vi "G#Object_RegisterExternalCreateProcessCallers.vi"(1 "Action":T1(ring), 5 "error in (no error)":errorcluster) -> (15 "StopExternalCreate?":bool, 19 "error out":errorcluster)   [LabVIEW 2020, in "G#Object.lvclass"]
doc: "Registers or deregister top-level callesrs."
uses:
  G#Object.lvclass
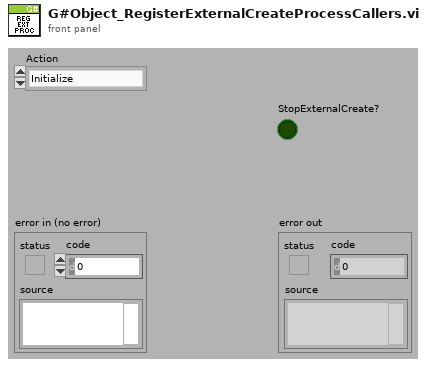
[diagram p1: front panel]
types:
  T1 = enum16{"Initialize", "Register", "Unregister", "Clear"}
  T2 = enum32{"Bad", "Idle", "Run top level", "Running"}
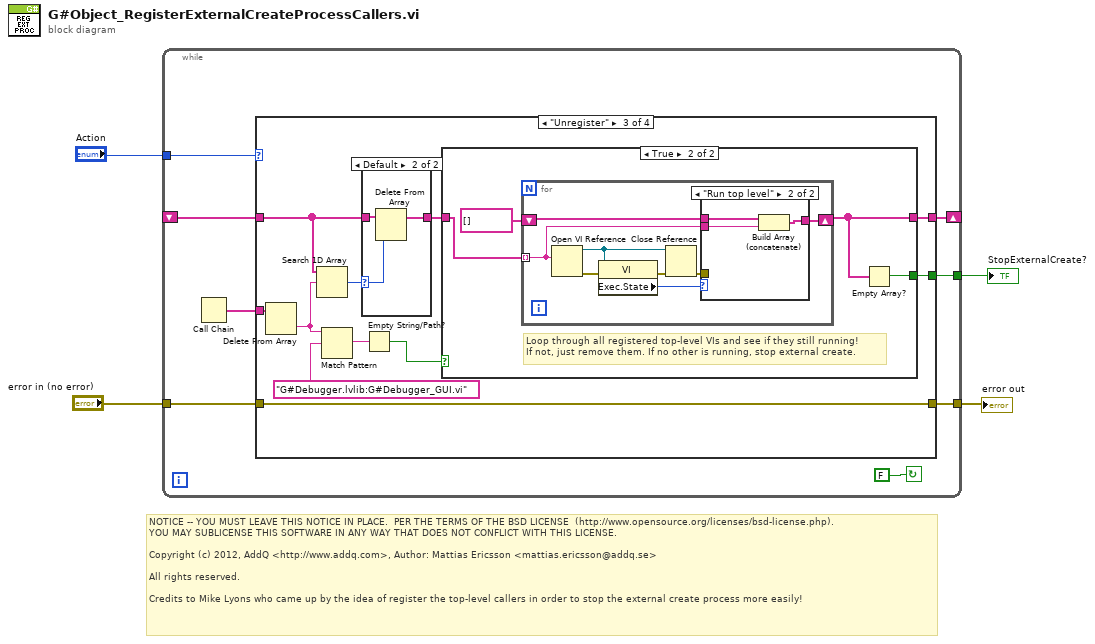
[diagram p0: block diagram]
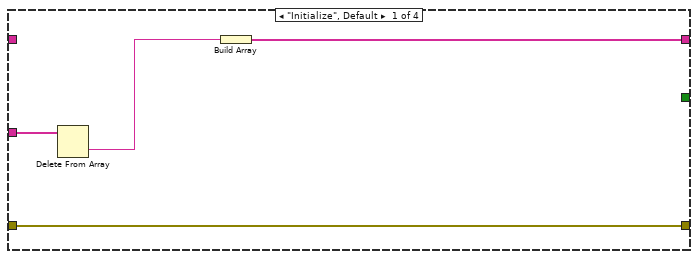
[diagram p2: hidden frame]
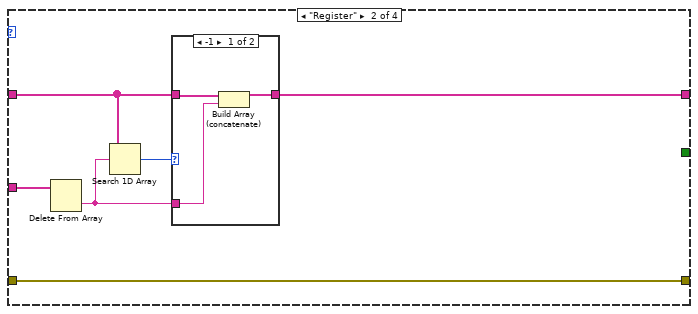
[diagram p3: hidden frame]
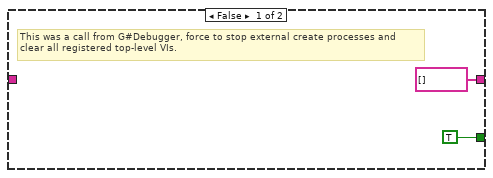
[diagram p5: hidden frame]
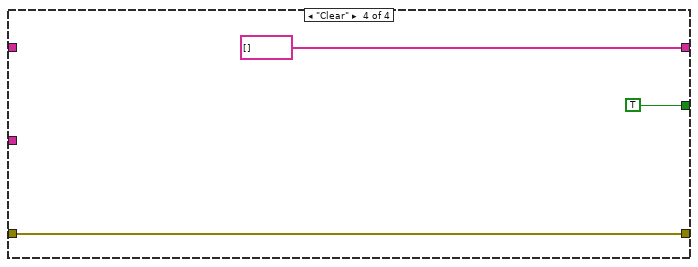
[diagram p8: hidden frame]
diagram:
  # "NOTICE -- YOU MUST LEAVE THIS NOTICE IN PLACE.  PER THE TERMS OF THE BSD LICENSE  (http://www.opensource.org/licenses/bsd-license.php).\nYOU MAY SUBLICENSE THIS SOFTWARE IN ANY WAY THAT DOES NOT CONFLICT WITH THIS LICENSE.\n\nCopyright (c) 2012, AddQ <http://www.addq.com>, Author: Mattias Ericsson <mattias.ericsson@addq.se>\n\nAll rights reserved.\n\nCredits to Mike Lyons who came up by the idea of register the top-level callers in order to stop the external create process more easily!"
  n1 = while {
    tunnel: "error in (no error)" -> [w11]
    tunnel: "Action" -> [w12]
    shift-right: [w8] -> _
    shift-left: _ -> [w6]
    tunnel: [w7] -> w2
    tunnel: [w5] -> w1
    stop <- FALSE continue-if-true
    n2 = Call Chain() -> (call chain=w9:string[])
    n3 = case shown="\"Unregister\"" w12 {
      tunnel: w11 -> [w13 w17 w33 w61]
      tunnel: w9 -> [w16 w22 w37 _]
      tunnel: [w15 w19 w31 string[] []] -> w8
      tunnel: [w13 w17 w33 w61] -> w7
      tunnel: w6 -> [_ w20 w35 _]
      tunnel: [_ _ w32 TRUE] -> w5
      frame "Initialize", Default {
        n4 = Delete From Array(array=w16) -> (deleted portion=w14:string)  [unwired: 2 in, 1 out]
        n5 = Build Array(w14) -> (w15:string[])
      }
      frame "Register" {
        n6 = Delete From Array(array=w22) -> (deleted portion=w18:string)  [unwired: 2 in, 1 out]
        n7 = Search 1D Array(1D array=w20, element=w18) -> (index of element=w21:i32)  [unwired: 1 in]
        n8 = case shown="-1" w21 {
          tunnel: w20 -> [w25 w26]
          tunnel: [w23 w26] -> w19
          tunnel: w18 -> [w24 _]
          frame -1 {
            n9 = Build Array (concatenate)(w25, w24) -> (w23:string[])
          }
          frame Default {
          }
        }
      }
      frame "Unregister" {
        n10 = Delete From Array(array=w37) -> (deleted portion=w30:string)  [unwired: 2 in, 1 out]
        n11 = Search 1D Array(1D array=w35, element=w30) -> (index of element=w36:i32)  [unwired: 1 in]
        n12 = Match Pattern(string=w30, regular expression="G#Debugger.lvlib:G#Debugger_GUI.vi") -> (match substring=w28:string)  [unwired: 1 in, 3 out]
        n13 = case shown="Default" w36 {
          selector: w36 -> [_ w57]
          tunnel: w35 -> [w56 w59]
          tunnel: [w56 w58] -> w34
          frame -1 {
          }
          frame Default {
            n14 = Delete From Array(array=w59, index=w57) -> (array with subset deleted=w58:string[])  [unwired: 1 in, 1 out]
          }
        }
        n15 = Empty String/Path?(string/path=w28) -> (empty?=w27:bool)
        n16 = case shown="True" w27 {
          tunnel: w34 -> [_ w43]
          tunnel: [TRUE w41] -> w32
          tunnel: [string[] [] w40] -> w31
          frame False {
            # "This was a call from G#Debugger, force to stop external create processes and\nclear all registered top-level VIs."
          }
          frame True {
            # "Loop through all registered top-level VIs and see if they still running!\nIf not, just remove them. If no other is running, stop external create."
            n17 = for {
              tunnel: w43 -> [w47] mode=indexing
              shift-right: [w45] -> w40
              shift-left: string[] [] -> [w46]
              n18 = Open VI Reference(vi path=w47) -> (vi reference=w48:refnum<vi>, error out=w51:errorcluster)  [unwired: 5 in]
              n19 = property class="VI"(reference=w48, error in=w51) -> (error out=w49:errorcluster, "Exec.State"=w50:T2)  [unwired: 1 out]
              n20 = Close Reference(reference=w48, error in (no error)=w49) -> (error out=w44:errorcluster)
              n21 = case shown="\"Run top level\"" w50 {
                tunnel: w47 -> [_ w54]
                tunnel: w46 -> [w52 w55]
                tunnel: [w52 w53] -> w45
                tunnel: w44 -> [_ _]
                frame Default {
                }
                frame "Run top level" {
                  n22 = Build Array (concatenate)(w55, w54) -> (w53:string[])
                }
              }
            }
            n23 = Empty Array?(array=w40) -> (empty?=w41:bool)
          }
        }
      }
      frame "Clear" {
      }
    }
  }
  "error out" <- w2
  "StopExternalCreate?" <- w1
